vi "PS_LCR_cal_probe.vi"(10 "Lower Voltge Limit":dbl=1.2, 11 "Upper Voltage Limit":dbl=4.0) -> (0 "Min":dbl, 1 "XY Graph":cluster{"Y":dbl[], "Y":dbl[]}[](graph)=[{"Y"=[0.0, 0.05, 0.1, 0.15, 0.2, 0.25, 0.3, 0.35, 0.4, 0.45, 0.5, 0.55, 0.6, 0.65, 0.7, 0.75, 0.8, 0.85, 0.9, 0.95, 1.0, 1.05, 1.1, 1.15, 1.2, 1.25, 1.3, 1.35, 1.4, 1.45, 1.5, 1.55, 1.6, 1.65, 1.7, 1.75, 1.8, 1.85, 1.9, 1.95, 2.0, 2.05, 2.1, 2.15, 2.2, 2.25, 2.3, 2.35, 2.4, 2.45, 2.5, 2.55, 2.6, 2.65, 2.7, 2.75, 2.8, 2.85, 2.9, 2.95, 3.0, 3.05, 3.1, 3.15, 3.2, 3.25, 3.3, 3.35, 3.4, 3.45, 3.5, 3.55, 3.6, 3.65, 3.7, 3.75, 3.8, 3.85, 3.9, 3.95, 4.0, 4.05, 4.1, 4.15, 4.2, 4.25, 4.3, 4.35, 4.4, 4.45, 4.5, 4.55, 4.6, 4.65, 4.7, 4.75, 4.8, 4.85, 4.9, 4.95, 5.0, 5.05], "Y"=[1.5298757135269085, 1.5328388976296985, 1.5293925856704482, 1.5345781578612852, 1.5339661959375244, 1.53018169447358, 1.5265743399104366, 1.5220007296691076, 1.51427068423586, 1.5063957004884947, 1.4997124321084379, 1.4819977450237825, 1.4447163815532993, 1.3573024588883174, 1.161603516393886, 0.820918029268634, 0.4199061821541399, 0.153622585843183, 0.15030511317271325, 0.43882866711630325, 0.9999006895515649, 1.7411958476019447, 2.5304981523045864, 3.255995414422078, 3.818694517751893, 4.165918458818913, 4.28151481082073, 4.198819455810404, 3.959059256056534, 3.6098544367966032, 3.1979556371752222, 2.7795023464614927, 2.353174058815591, 1.9588288800544416, 1.6140365864269837, 1.3070571708940657, 1.0370854125367381, 0.8146051627749571, 0.6324661084613775, 0.488896759796258, 0.3677123343585585, 0.27295498563700904, 0.2089245346149273, 0.1557966576810819, 0.11780676597356136, 0.09493875253211967, 0.08471256374939808, 0.07883451829497443, 0.07988129347656164, 0.08679000994821919, 0.1060506744395145, 0.11840262266212312, 0.14189870211324745, 0.16217393518736928, 0.18887475937212259, 0.21549506349261563, 0.24541673756696256, 0.27099026846865953, 0.29912437444837736, 0.32951307523590956, 0.3613189505652336, 0.3922229898377022, 0.4230787177962361, 0.44779873039006196, 0.4836145678075603, 0.509687339034607, 0.5342946249192798, 0.5705774896484697, 0.6011594528745015, 0.6259599926645998, 0.6571217110122272, 0.6779283991150254, 0.7090740151905816, 0.7342932688254709, 0.7632809176513753, 0.787839898681874, 0.815201020034375, 0.8366357778752933, 0.8612269695320995, 0.891003730987698, 0.9074461724203882, 0.9323916595874564, 0.957933004817351, 0.981493527508089, 1.0035080424099714, 1.0244435728298853, 1.046007169575612, 1.0641888732873335, 1.082000179455684, 1.1046749711119777, 1.124096703595656, 1.14831750481961, 1.1598159438564613, 1.180815894520082, 1.2004630880208707, 1.2108342296260255, 1.2341531943794966, 1.245104089613326, 1.2719659918665696, 1.2829813044791825, 1.3021775805287772, 1.3143201915840468]}], 2 "Min Voltage":dbl, 3 "Max Voltage":dbl)   [LabVIEW 2011]
uses:
  PS_Global.vi
  <vilib>/Instr/_visa.llb/VISA Configure Serial Port (Instr).vi
  <vilib>/Analysis/NI_AALBase.lvlib
panel:
  in  "Stop at Voltage":dbl=5.0
  in  "Number of Points":dbl=100.0
  out "Max":dbl
  out "Waveform Chart 2":dbl(graph)
  in  "baud rate":u32=115200
  out "Waveform Chart":dbl(graph)
  out "Signal Mean":dbl format="%0.2f"
  out "Voltage 2 Setpoint":dbl
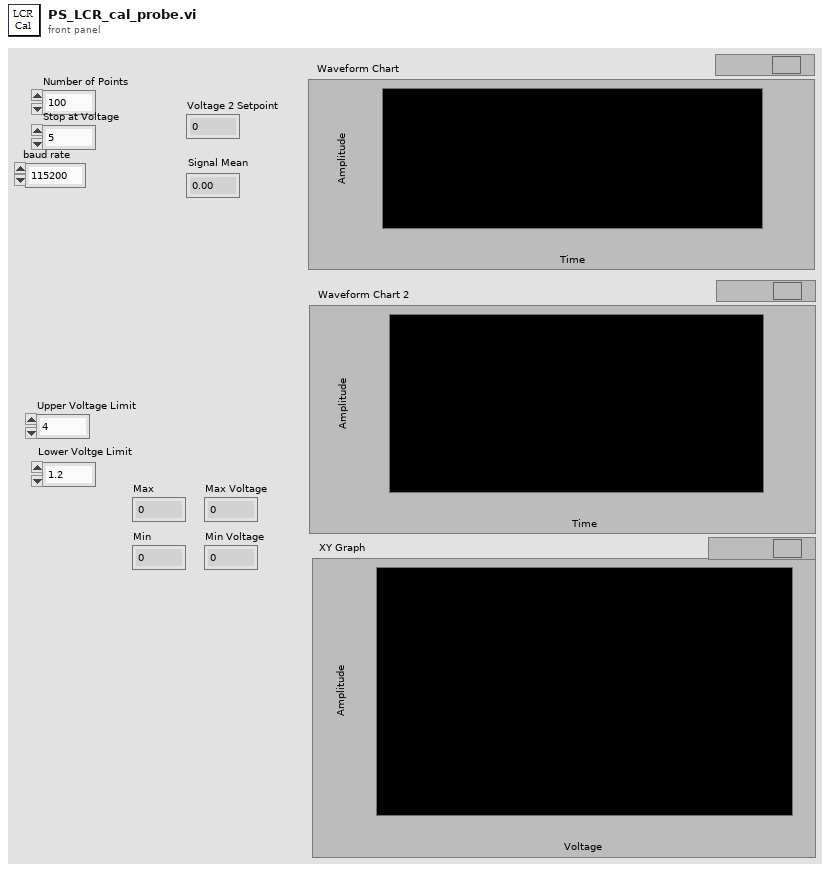
[diagram p1: front panel]
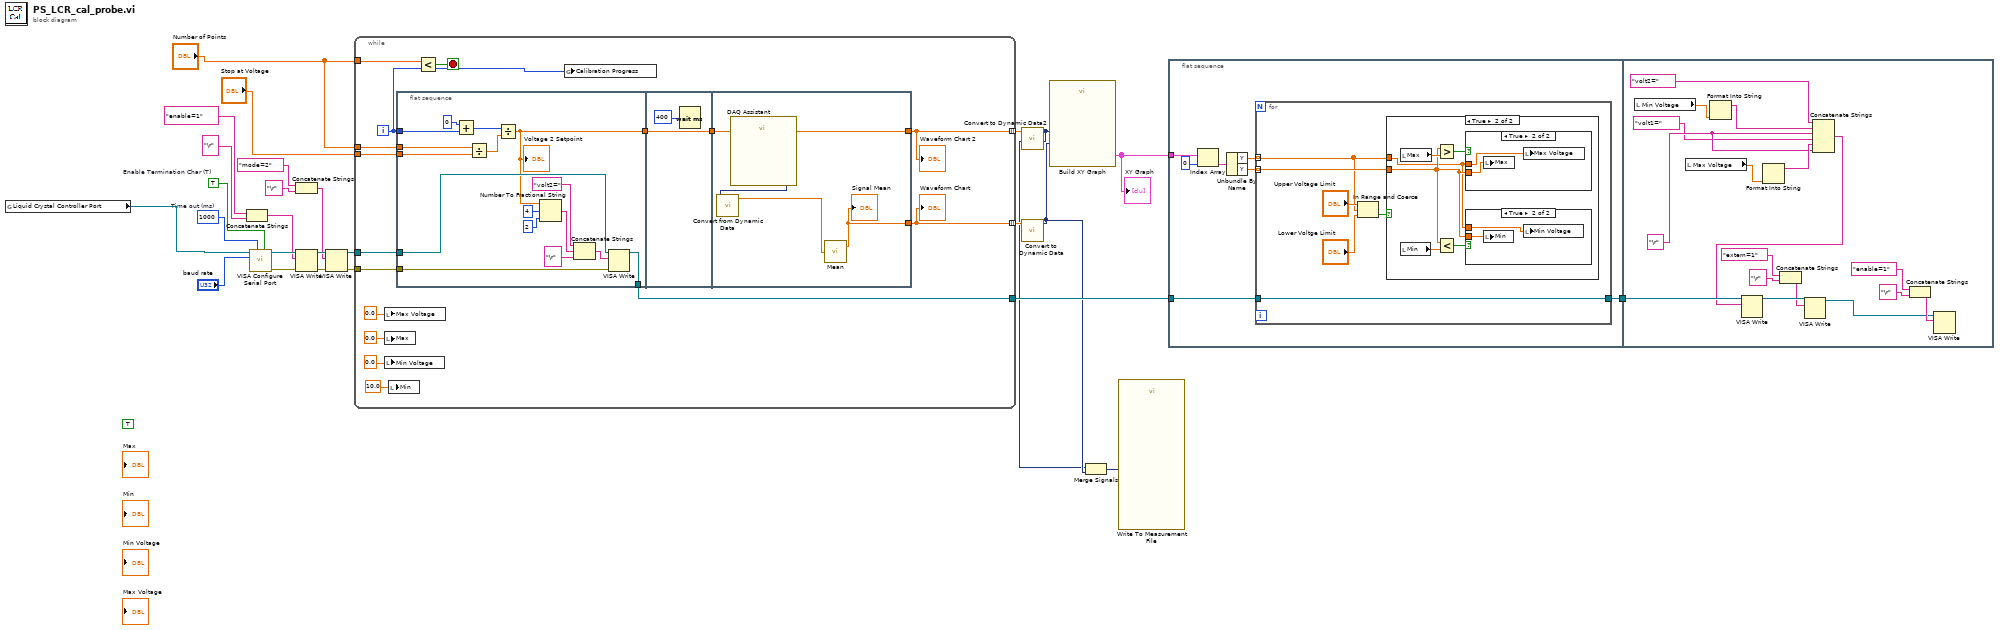
[diagram p0: block diagram]
diagram:
  (unwired) TRUE
  w22 = TRUE  # Enable Termination Char (T)
  w25 = 1000  # Time out (ms)
  n1 = global read "PS_Global.vi" "Liquid Crystal Controller Port"() -> (w3:refnum<visa-resource-name>)
  n2 = Concatenate Strings("enable=1", "\r") -> (w19:string)
  n3 = call-poly "VISA Configure Serial Port"("VISA resource name"=w3, "timeout (10sec)"=w25, "Enable Termination\nChar (T)"=w22, "baud rate (9600)"="baud rate") -> ("VISA resource name out"=w24:refnum<visa-resource-name>, "error out"=w23:errorcluster)  [unwired: 10 in]
  n4 = Concatenate Strings("mode=2" ("write buffer"), "\r") -> (w15:string)
  n5 = VISA Write(VISA resource name=w24, write buffer=w19, error in (no error)=w23) -> (VISA resource name out=w16:refnum<visa-resource-name>, error out=w14:errorcluster)  [unwired: 1 out]
  n6 = VISA Write(VISA resource name=w16, write buffer=w15, error in (no error)=w14) -> (VISA resource name out=w12:refnum<visa-resource-name>, error out=w13:errorcluster)  [unwired: 1 out]
  n7 = while {
    tunnel: w12 -> [w41]
    tunnel: w13 -> [w40]
    tunnel: [w37] -> w11 mode=indexing
    tunnel: [w36] -> w10 mode=indexing
    tunnel: [w31] -> w8
    tunnel: "Number of Points" -> [w29]
    tunnel: "Number of Points" -> [w28]
    tunnel: "Stop at Voltage" -> [w27]
    i -> [w30]
    stop <- w42 stop-if-true
    n8 = local write "Max Voltage"(0.0 ("Max Voltage")) -> ()
    n9 = local write "Max"(0.0 ("Max")) -> ()
    n10 = local write "Min Voltage"(0.0 ("Min Voltage")) -> ()
    n11 = local write "Min"(10.0 ("Min")) -> ()
    n12 = flat-sequence {
      tunnel: w30 -> [w50]
      tunnel: w41 -> [w56]
      tunnel: w40 -> [w55]
      tunnel: [w47] -> w38
      tunnel: [w46] -> w31
      tunnel: w28 -> [w44]
      tunnel: w27 -> [w43]
      tunnel: [w59] -> w39
      tunnel: w38 -> [w59]
      tunnel: w39 -> [w62]
      tunnel: [w63] -> w37
      tunnel: [w62] -> w36
      frame #0 {
        n13 = Add(x=0, y=w50) -> (x+y=w51:i32)
        n14 = Divide(x=w44, y=w43) -> (x/y=w45:dbl)
        n15 = Divide(x=w51, y=w45) -> (x/y=w47:dbl)
        "Voltage 2 Setpoint" <- w47
        n16 = Number To Fractional String(number=w47, width (-)=i16 4, precision (6)=i16 2) -> (F-format string=w54:string)  [unwired: 1 in]
        n17 = Concatenate Strings("volt2=" ("string"), w54, "\r") -> (w57:string)
        n18 = VISA Write(VISA resource name=w56, write buffer=w57, error in (no error)=w55) -> (VISA resource name out=w46:refnum<visa-resource-name>)  [unwired: 2 out]
      }
      frame #1 {
        n19 = Wait (ms)(milliseconds to wait=u32 400) -> ()  [unwired: 1 out]
      }
      frame #2 {
        n20 = call "DAQ Assistant"() -> ("data"=w64:dynamicdata)  [unwired: 17 in, 2 out]
        n21 = call "Convert from Dynamic Data"("Dynamic Data Type"=w64) -> ("Array"=w61:dbl[])  [unwired: 3 in]
        n22 = call <vilib>:"Mean.vi"("X"=w61) -> ("mean"=w63:dbl)  [unwired: 1 out]
        "Signal Mean" <- w63
      }
    }
    n23 = Less?(x=w29, y=w30) -> (x < y?=w42:bool)
    n24 = global write "PS_Global.vi" "Calibration Progress"(w30) -> ()
    "Waveform Chart" <- w37
    "Waveform Chart 2" <- w36
  }
  n25 = call "Convert to Dynamic Data2"("Array"=w10) -> ("Dynamic Data Type"=w5:dynamicdata)  [unwired: 3 in]
  n26 = call "Convert to Dynamic Data"("Array"=w11) -> ("Dynamic Data Type"=w6:dynamicdata)  [unwired: 3 in]
  n27 = call "Build XY Graph"("Y Input"=w6, "X Input"=w5) -> ("XY Graph"=w9:cluster{"Y":dbl[], "Y":dbl[]}[])  [unwired: 3 in, 6 out]
  "XY Graph" <- w9
  n28 = Merge Signals(w5, w6) -> (w4:dynamicdata)
  n29 = call "Write To Measurement File"("Signals"=w4) -> ()  [unwired: 16 in, 3 out]
  n30 = flat-sequence {
    tunnel: w9 -> [w71]
    tunnel: w8 -> [w66]
    tunnel: [w65] -> w7
    tunnel: w7 -> [w104]
    frame #0 {
      n31 = Index Array(array=w71, index=0) -> (element=w69:cluster{"Y":dbl[], "Y":dbl[]})
      n32 = Unbundle By Name(w69) -> ("Y"=w68:dbl[], "Y"=w67:dbl[])
      n33 = for {
        tunnel: w68 -> [w73] mode=indexing
        tunnel: w67 -> [w74] mode=indexing
        tunnel: w66 -> [w72]
        tunnel: [w72] -> w65
        n34 = In Range and Coerce(upper limit="Upper Voltage Limit", x=w73, lower limit="Lower Voltge Limit") -> (In Range?=w77:bool)  [unwired: 1 out]
        n35 = case shown="True" w77 {
          tunnel: w74 -> [_ w79]
          tunnel: w73 -> [_ w78]
          frame False {
          }
          frame True {
            n36 = local read "Max"() -> (w81:dbl)
            n37 = local read "Min"() -> (w82:dbl)
            n38 = Greater?(x=w79, y=w81) -> (0:w80:bool)
            n39 = Less?(x=w79, y=w82) -> (x < y?=w83:bool)
            n40 = case shown="True" w80 {
              tunnel: w79 -> [_ w87]
              tunnel: w78 -> [_ w86]
              frame False {
              }
              frame True {
                n41 = local write "Max"(w87) -> ()
                n42 = local write "Max Voltage"(w86) -> ()
              }
            }
            n43 = case shown="True" w83 {
              tunnel: w79 -> [_ w85]
              tunnel: w78 -> [_ w84]
              frame False {
              }
              frame True {
                n44 = local write "Min"(w85) -> ()
                n45 = local write "Min Voltage"(w84) -> ()
              }
            }
          }
        }
      }
    }
    frame #1 {
      w97 = "\r"
      n46 = local read "Min Voltage"() -> (w102:dbl)
      n47 = local read "Max Voltage"() -> (w99:dbl)
      n48 = Format Into String(w102) -> (resulting string=w100:string)  [unwired: 3 in, 1 out]
      n49 = Format Into String(w99) -> (resulting string=w98:string)  [unwired: 3 in, 1 out]
      n50 = Concatenate Strings("extern=1" ("write buffer"), "\r") -> (w92:string)
      n51 = Concatenate Strings("volt2=" ("write buffer"), w100, w97, "volt1=" ("write buffer"), w98, w97) -> (w103:string)
      n52 = VISA Write(VISA resource name=w104, write buffer=w103) -> (VISA resource name out=w95:refnum<visa-resource-name>)  [unwired: 1 in, 2 out]
      n53 = VISA Write(VISA resource name=w95, write buffer=w92) -> (VISA resource name out=w88:refnum<visa-resource-name>)  [unwired: 1 in, 2 out]
      n54 = Concatenate Strings("enable=1" ("write buffer"), "\r") -> (w91:string)
      n55 = VISA Write(VISA resource name=w88, write buffer=w91) -> ()  [unwired: 1 in, 3 out]
    }
  }
